vi "AMZ_S3_URLEncode String.vi"(4 "Unescaped string in":string) -> (1 "Escaped string out":string)   [LabVIEW 2015, in "LV Interface for Amazon S3.lvlib"]
doc: "Percent-encodes URL-unsafe characters."
uses:
  LV Interface for Amazon S3.lvlib
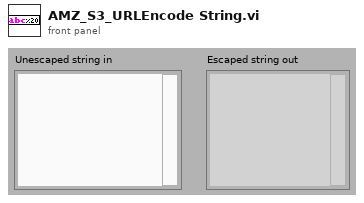
[diagram p1: front panel]
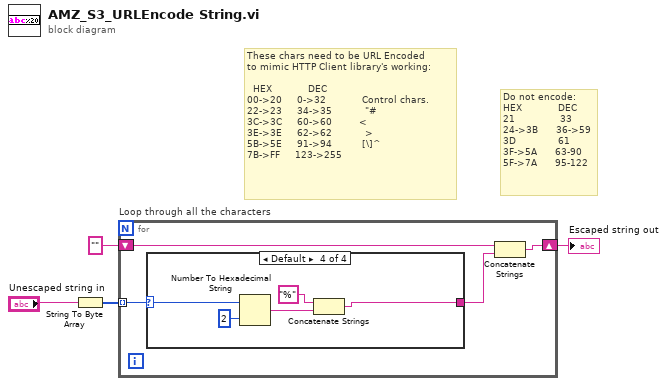
[diagram p0: block diagram]
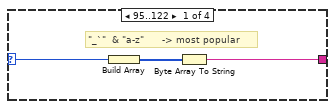
[diagram p2: hidden frame]
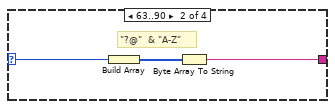
[diagram p3: hidden frame]
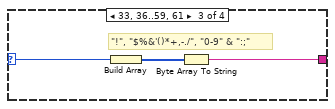
[diagram p4: hidden frame]
diagram:
  # "Do not encode:\nHEX            DEC\n21               33\n24->3B      36->59\n3D              61\n3F->5A      63-90\n5F->7A      95-122"
  # "These chars need to be URL Encoded\nto mimic HTTP Client library's working:\n\n  HEX            DEC\n00->20     0->32            Control chars.\n22->23     34->35           \"# \n3C->3C     60->60         <\n3E->3E     62->62           >\n5B->5E     91->94          [\\]^\n7B->FF     123->255"
  n1 = String To Byte Array(string="Unescaped string in") -> (unsigned byte array=w2:u8[])
  n2 = for "Loop through all the characters" {
    shift-right: [w5] -> w4
    shift-left: "" -> [w6]
    tunnel: w2 -> [w8] mode=indexing
    n3 = case shown="Default" w8 {
      selector: w8 -> [w11 w14 w16 w22]
      tunnel: [w9 w12 w15 w18] -> w7
      frame 95..122 {
        # "\"_`\"  & \"a-z\"      -> most popular"
        n4 = Build Array(w11) -> (w10:u8[])
        n5 = Byte Array To String(unsigned byte array=w10) -> (string=w9:string)
      }
      frame 63..90 {
        # "\"?@\"  & \"A-Z\""
        n6 = Build Array(w14) -> (w13:u8[])
        n7 = Byte Array To String(unsigned byte array=w13) -> (string=w12:string)
      }
      frame 33, 36..59, 61 {
        # "\"!\", \"$%&'()*+,-./\", \"0-9\" & \":;\""
        n8 = Build Array(w16) -> (w17:u8[])
        n9 = Byte Array To String(unsigned byte array=w17) -> (string=w15:string)
      }
      frame Default {
        n10 = Number To Hexadecimal String(1:i16 2 ("width (-)"), 2:w22) -> (0:w20:string)
        n11 = Concatenate Strings("%" ("string"), w20) -> (w18:string)
      }
    }
    n12 = Concatenate Strings(w6, w7) -> (w5:string)
  }
  "Escaped string out" <- w4
